vi "Evaluate Save Test Executive.vi"(8 "error in (no error)":errorcluster, 10 "Create Test Executive":T1, 11 "Test Executive Builder Model in":refnum<class "Test Executive Builder Model.lvclass">) -> (0 "error out":errorcluster, 3 "Test Executive Builder Model out":refnum<class "Test Executive Builder Model.lvclass">)   [LabVIEW 2017, in "Test Executive Builder Model.lvclass"]
uses:
  <vilib>/gpm_packages/@cs/Test-executive-builder/Source/Test Executive Builder Model/Test Executive Builder Model/Test Executive Builder Model.lvclass
  <vilib>/gpm_packages/@cs/Test-executive-builder/Source/Application Dependencies/Create Test Executive.ctl
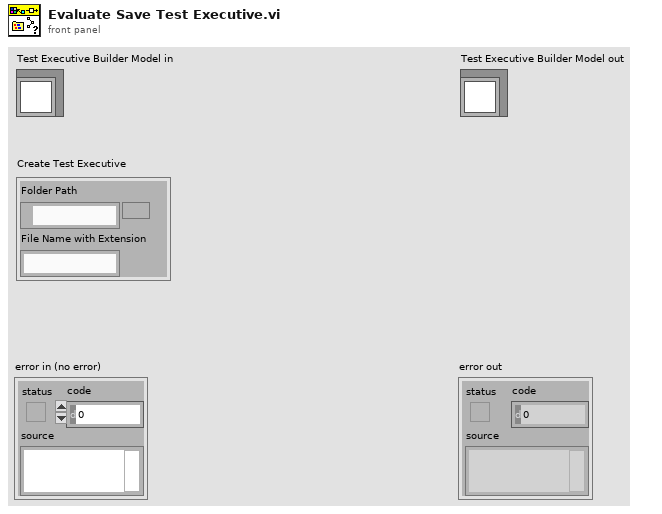
[diagram p1: front panel]
types:
  T1 = typedef "Create Test Executive.ctl" = cluster{"Folder Path":path, "File Name with Extension":string}
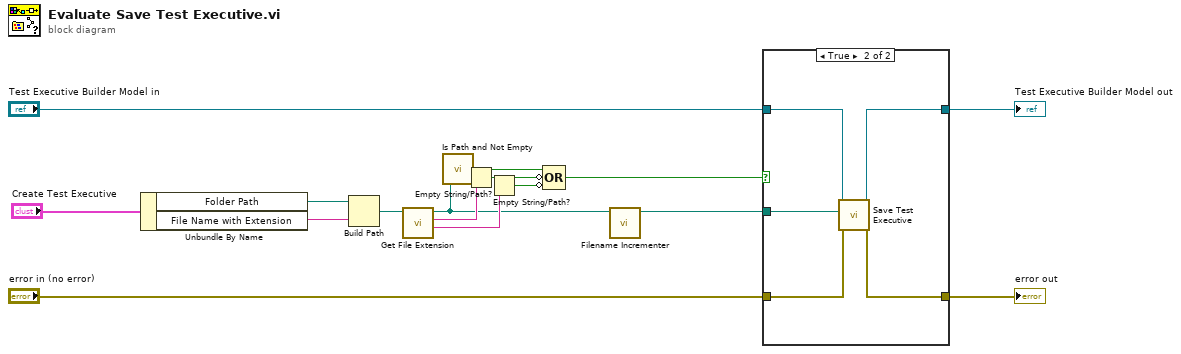
[diagram p0: block diagram]
diagram:
  n1 = Unbundle By Name("Create Test Executive") -> ("Folder Path"=w3:path, "File Name with Extension"=w4:string)
  n2 = Build Path(base path=w3, name or relative path=w4) -> (appended path=w16:path)
  n3 = call <vilib>:"Get File Extension.vi"("file"=w16) -> ("filename without extension"=w12:string, "lowercase file extension"=w14:string, "dup file"=w2:path)  [unwired: 6 in, 2 out]
  n4 = call <vilib>:"Is Path and Not Empty.vi"("path"=w2) -> ("Is Path and Not Empty?"=w15:bool)  [unwired: 4 in]
  n5 = Empty String/Path?(string/path=w14) -> (empty?=w13:bool)
  n6 = Empty String/Path?(string/path=w12) -> (empty?=w11:bool)
  n7 = Compound Arithmetic op=OR(w15, invert w13, invert w11) -> (w8:bool)
  n8 = call <vilib>:"Filename Incrementer.vi"("File Path"=w2) -> ("File Path out"=w1:path)  [unwired: 10 in]
  n9 = case shown="True" w8 {
    tunnel: "Test Executive Builder Model in" -> [w18 w23]
    tunnel: [w18 w22] -> w9
    tunnel: "error in (no error)" -> [w17 w21]
    tunnel: [w17 w20] -> w6
    tunnel: w1 -> [_ w19]
    frame False {
    }
    frame True {
      n10 = call-dynamic "Save Test Executive.vi"("error in (no error)"=w21, "Path"=w19, "Test Executive Builder Model in"=w23) -> ("error out"=w20:errorcluster, "Test Executive Builder Model out"=w22:refnum<class "Test Executive Builder Model.lvclass">)  [unwired: 7 in]
    }
  }
  "error out" <- w6
  "Test Executive Builder Model out" <- w9
